vi "T1T2占空比副本.vi"() -> ()   [LabVIEW 2020]
uses:
  <vilib>/DAQmx/read.llb/DAQmx Read (Counter 1D DBL 1Chan NSamp).vi
  Global_Variable/Global.vi
  <vilib>/DAQmx/create/channels.llb/DAQmx Create Channel (CI-Period).vi
  <vilib>/DAQmx/configure/timing.llb/DAQmx Timing (Implicit).vi
  <vilib>/DAQmx/miscellaneous.llb/DAQmx Fill In Error Info.vi
  <userlib>/_MGI/1D Array/MGI Average/MGI Average (DBL[]).vi
  <vilib>/DAQmx/create/channels.llb/DAQmx Create Channel (CI-Pulse Width).vi
  <resource>/objmgr/daqmx.rc
panel:
  out "T2":dbl
  out "T2周期":dbl
  out "T1周期":dbl
  out "T1":dbl
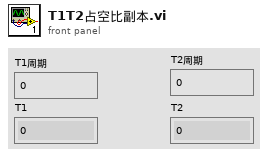
[diagram p1: front panel]
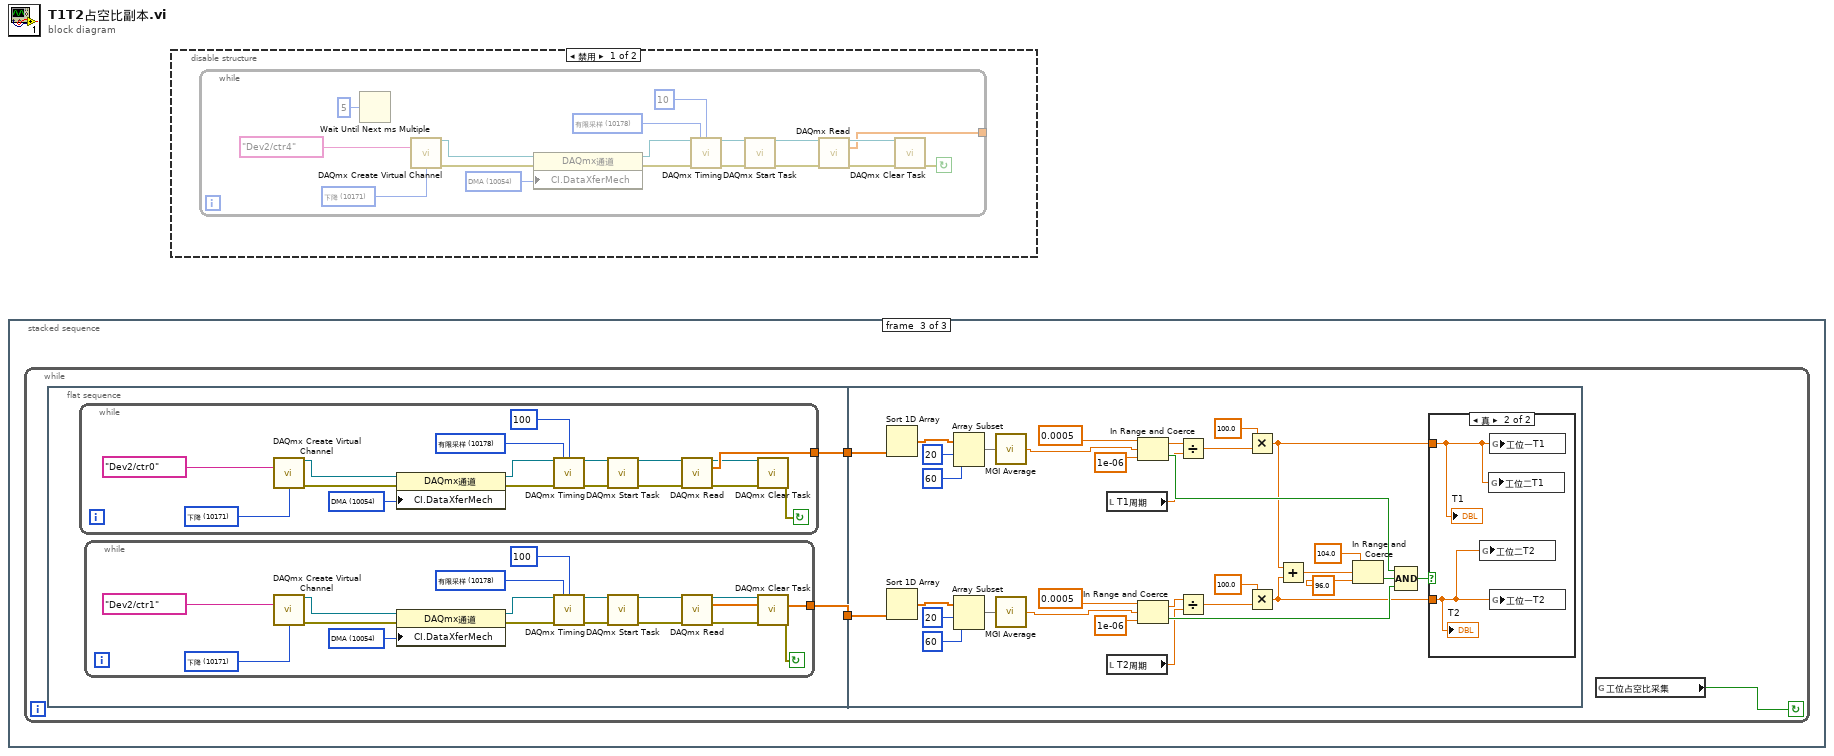
[diagram p0: block diagram]
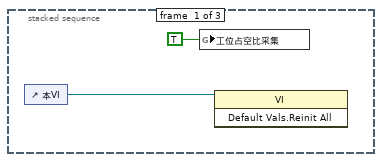
[diagram p3: hidden frame]
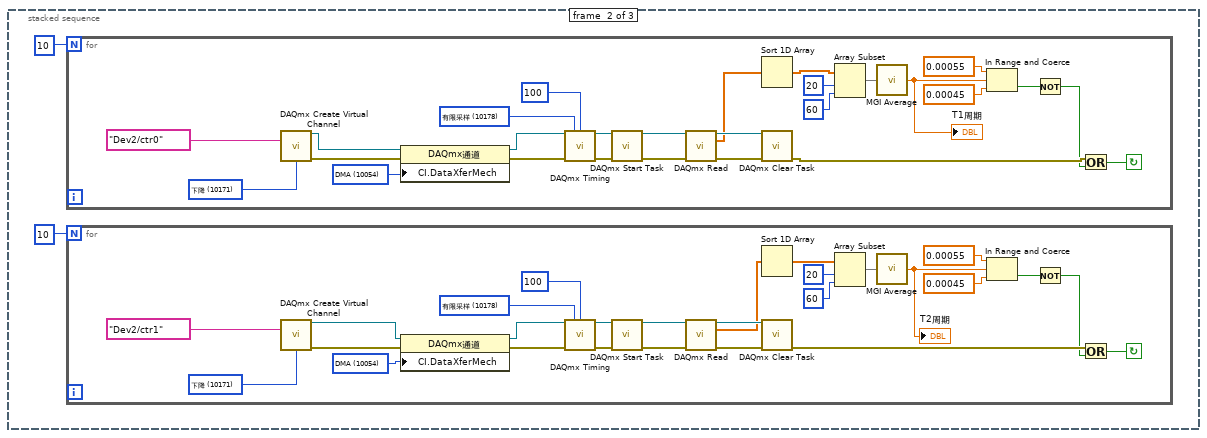
[diagram p4: hidden frame]
diagram:
  n1 = stacked-sequence {
    frame #0 {
      n2 = control-ref of="本VI"() -> (w2:refnum<vi>)
      n3 = global write "Global.vi" "工位占空比采集"(TRUE ("工位一占空比采集")) -> ()
      n4 = invoke class="VI" method="Default Vals.Reinit All"(reference=w2) -> ()  [unwired: 2 in, 3 out]
    }
    frame #1 {
      n5 = for {
        N: 10 -> [_]
        stop <- w32 continue-if-true
        w45 = 10054 items=["DMA"=10054, "中断"=10204, "程序控制I/O"=10264, "USB Bulk"=12590] ("CI.DataXferMech")
        w49 = 10178 items=["有限采样"=10178, "连续采样"=10123, "硬件定时单点"=12522] ("sample mode")
        w58 = 10171 items=["上升"=10280, "下降"=10171] ("starting edge")
        n6 = call-poly <vilib>:"DAQmx Create Virtual Channel.vi"("counter"=tag "Dev2/ctr0", "starting edge"=w58) -> ("task out"=w57:refnum<k21>, "error out"=w47:errorcluster)  [unwired: 12 in]
        n7 = property class="DAQmx通道"(reference=w57, error in=w47, "CI.DataXferMech"=w45) -> (reference out=w48:refnum<k21>, error out=w46:errorcluster)
        n8 = call-poly <vilib>:"DAQmx Timing.vi"("task/channels in"=w48, "sample mode"=w49, "samples per channel"=100, "error in"=w46) -> ("task out"=w56:refnum<k21>, "error out"=w55:errorcluster)  [unwired: 10 in]
        n9 = call <vilib>:"DAQmx Start Task.vi"("task/channels in"=w56, "error in"=w55) -> ("task out"=w54:refnum<k21>, "error out"=w53:errorcluster)  [unwired: 12 in]
        n10 = call-poly <vilib>:"DAQmx Read.vi"("task/channels in"=w54, "error in"=w53) -> ("task out"=w51:refnum<k21>, "data"=w39:dbl[], "error out"=w52:errorcluster)  [unwired: 11 in]
        n11 = Sort 1D Array(array=w39) -> (sorted array=w42:dbl[])
        n12 = call <vilib>:"DAQmx Clear Task.vi"("task in"=w51, "error in"=w52) -> ("error out"=w34:errorcluster)  [unwired: 13 in]
        n13 = Array Subset(array=w42, index=20 ("索引"), length=60 ("长度")) -> (w43:dbl[])
        n14 = call-poly <userlib>:"MGI Average.vi"("Double[]"=w43) -> ("Average"=w38:dbl)  [unwired: 1 in]
        "T1周期" <- w38
        n15 = In Range and Coerce(upper limit=0.00055 ("上限"), x=w38, lower limit=0.00045 ("上限")) -> (In Range?=w35:bool)  [unwired: 1 out]
        n16 = Not(x=w35) -> (.not. x?=w33:bool)
        n17 = Or(x=w34, y=w33) -> (x .or. y?=w32:bool)
      }
      n18 = for {
        N: 10 -> [_]
        stop <- w5 continue-if-true
        w18 = 10054 items=["DMA"=10054, "中断"=10204, "程序控制I/O"=10264, "USB Bulk"=12590] ("CI.DataXferMech")
        w22 = 10178 items=["有限采样"=10178, "连续采样"=10123, "硬件定时单点"=12522] ("sample mode")
        w31 = 10171 items=["上升"=10280, "下降"=10171] ("starting edge")
        n19 = call-poly <vilib>:"DAQmx Create Virtual Channel.vi"("counter"=tag "Dev2/ctr1", "starting edge"=w31) -> ("task out"=w30:refnum<k21>, "error out"=w20:errorcluster)  [unwired: 12 in]
        n20 = property class="DAQmx通道"(reference=w30, error in=w20, "CI.DataXferMech"=w18) -> (reference out=w21:refnum<k21>, error out=w19:errorcluster)
        n21 = call-poly <vilib>:"DAQmx Timing.vi"("task/channels in"=w21, "sample mode"=w22, "samples per channel"=100, "error in"=w19) -> ("task out"=w29:refnum<k21>, "error out"=w28:errorcluster)  [unwired: 10 in]
        n22 = call <vilib>:"DAQmx Start Task.vi"("task/channels in"=w29, "error in"=w28) -> ("task out"=w27:refnum<k21>, "error out"=w26:errorcluster)  [unwired: 12 in]
        n23 = call-poly <vilib>:"DAQmx Read.vi"("task/channels in"=w27, "error in"=w26) -> ("task out"=w24:refnum<k21>, "data"=w12:dbl[], "error out"=w25:errorcluster)  [unwired: 11 in]
        n24 = Sort 1D Array(array=w12) -> (sorted array=w16:dbl[])
        n25 = call <vilib>:"DAQmx Clear Task.vi"("task in"=w24, "error in"=w25) -> ("error out"=w8:errorcluster)  [unwired: 13 in]
        n26 = Array Subset(array=w16, index=20 ("索引"), length=60 ("长度")) -> (w15:dbl[])
        n27 = call-poly <userlib>:"MGI Average.vi"("Double[]"=w15) -> ("Average"=w9:dbl)  [unwired: 1 in]
        "T2周期" <- w9
        n28 = In Range and Coerce(upper limit=0.00055 ("上限"), x=w9, lower limit=0.00045 ("上限")) -> (In Range?=w7:bool)  [unwired: 1 out]
        n29 = Not(x=w7) -> (.not. x?=w6:bool)
        n30 = Or(x=w8, y=w6) -> (x .or. y?=w5:bool)
      }
    }
    frame #2 {
      n31 = while {
        stop <- w61 continue-if-true
        n32 = flat-sequence {
          tunnel: [w63] -> w60
          tunnel: [w62] -> w59
          tunnel: w60 -> [w98]
          tunnel: w59 -> [w101]
          frame #0 {
            n33 = while {
              tunnel: [w97] -> w63
              stop <- w81 continue-if-true
              w83 = 10054 items=["DMA"=10054, "中断"=10204, "程序控制I/O"=10264, "USB Bulk"=12590] ("CI.DataXferMech")
              w87 = 10178 items=["有限采样"=10178, "连续采样"=10123, "硬件定时单点"=12522] ("sample mode")
              w96 = 10171 items=["上升"=10280, "下降"=10171] ("starting edge")
              n34 = call-poly <vilib>:"DAQmx Create Virtual Channel.vi"("counter"=tag "Dev2/ctr0", "starting edge"=w96) -> ("task out"=w95:refnum<k21>, "error out"=w85:errorcluster)  [unwired: 12 in]
              n35 = property class="DAQmx通道"(reference=w95, error in=w85, "CI.DataXferMech"=w83) -> (reference out=w86:refnum<k21>, error out=w84:errorcluster)
              n36 = call-poly <vilib>:"DAQmx Timing.vi"("task/channels in"=w86, "sample mode"=w87, "samples per channel"=100, "error in"=w84) -> ("task out"=w94:refnum<k21>, "error out"=w93:errorcluster)  [unwired: 10 in]
              n37 = call <vilib>:"DAQmx Start Task.vi"("task/channels in"=w94, "error in"=w93) -> ("task out"=w92:refnum<k21>, "error out"=w91:errorcluster)  [unwired: 12 in]
              n38 = call-poly <vilib>:"DAQmx Read.vi"("task/channels in"=w92, "error in"=w91) -> ("task out"=w89:refnum<k21>, "data"=w97:dbl[], "error out"=w90:errorcluster)  [unwired: 11 in]
              n39 = call <vilib>:"DAQmx Clear Task.vi"("task in"=w89, "error in"=w90) -> ("error out"=w81:errorcluster)  [unwired: 13 in]
            }
            n40 = while {
              tunnel: [w80] -> w62
              stop <- w64 continue-if-true
              w66 = 10054 items=["DMA"=10054, "中断"=10204, "程序控制I/O"=10264, "USB Bulk"=12590] ("CI.DataXferMech")
              w70 = 10178 items=["有限采样"=10178, "连续采样"=10123, "硬件定时单点"=12522] ("sample mode")
              w79 = 10171 items=["上升"=10280, "下降"=10171] ("starting edge")
              n41 = call-poly <vilib>:"DAQmx Create Virtual Channel.vi"("counter"=tag "Dev2/ctr1", "starting edge"=w79) -> ("task out"=w78:refnum<k21>, "error out"=w68:errorcluster)  [unwired: 12 in]
              n42 = property class="DAQmx通道"(reference=w78, error in=w68, "CI.DataXferMech"=w66) -> (reference out=w69:refnum<k21>, error out=w67:errorcluster)
              n43 = call-poly <vilib>:"DAQmx Timing.vi"("task/channels in"=w69, "sample mode"=w70, "samples per channel"=100, "error in"=w67) -> ("task out"=w77:refnum<k21>, "error out"=w76:errorcluster)  [unwired: 10 in]
              n44 = call <vilib>:"DAQmx Start Task.vi"("task/channels in"=w77, "error in"=w76) -> ("task out"=w75:refnum<k21>, "error out"=w74:errorcluster)  [unwired: 12 in]
              n45 = call-poly <vilib>:"DAQmx Read.vi"("task/channels in"=w75, "error in"=w74) -> ("task out"=w72:refnum<k21>, "data"=w80:dbl[], "error out"=w73:errorcluster)  [unwired: 11 in]
              n46 = call <vilib>:"DAQmx Clear Task.vi"("task in"=w72, "error in"=w73) -> ("error out"=w64:errorcluster)  [unwired: 13 in]
            }
          }
          frame #1 {
            n47 = Sort 1D Array(array=w98) -> (sorted array=w112:dbl[])
            n48 = Sort 1D Array(array=w101) -> (sorted array=w115:dbl[])
            n49 = Array Subset(array=w112, index=20 ("索引"), length=60 ("长度")) -> (w113:dbl[])
            n50 = Array Subset(array=w115, index=20 ("索引"), length=60 ("长度")) -> (w114:dbl[])
            n51 = call-poly <userlib>:"MGI Average.vi"("Double[]"=w113) -> ("Average"=w116:dbl)  [unwired: 1 in]
            n52 = call-poly <userlib>:"MGI Average.vi"("Double[]"=w114) -> ("Average"=w118:dbl)  [unwired: 1 in]
            n53 = local read "T1周期"() -> (w121:dbl)
            n54 = local read "T2周期"() -> (w122:dbl)
            n55 = In Range and Coerce(upper limit=0.0005 ("上限"), x=w116, lower limit=1e-06 ("上限")) -> (coerced(x)=w117:dbl, In Range?=w127:bool)
            n56 = In Range and Coerce(upper limit=0.0005 ("上限"), x=w118, lower limit=1e-06 ("上限")) -> (coerced(x)=w119:dbl, In Range?=w128:bool)
            n57 = Divide(x=w117, y=w121) -> (x/y=w120:dbl)
            n58 = Divide(x=w119, y=w122) -> (x/y=w123:dbl)
            n59 = Multiply(x=100.0, y=w120) -> (x*y=w124:dbl)
            n60 = Multiply(x=100.0, y=w123) -> (x*y=w125:dbl)
            n61 = Add(x=w124, y=w125) -> (x+y=w126:dbl)
            n62 = In Range and Coerce(upper limit=104.0 ("上限"), x=w126, lower limit=96.0 ("下限")) -> (In Range?=w129:bool)  [unwired: 1 out]
            n63 = Compound Arithmetic op=AND ("复合运算")(w127, w129, w128) -> (w130:bool)
            n64 = case shown="真" w130 {
              tunnel: w124 -> [_ w132]
              tunnel: w125 -> [_ w131]
              frame False {
              }
              frame True {
                n65 = global write "Global.vi" "工位二T2"(w131) -> ()
                n66 = global write "Global.vi" "工位二T1"(w132) -> ()
                n67 = global write "Global.vi" "工位一T1"(w132) -> ()
                n68 = global write "Global.vi" "工位一T2"(w131) -> ()
                "T1" <- w132
                "T2" <- w131
              }
            }
          }
        }
        n69 = global read "Global.vi" "工位占空比采集"() -> (w61:bool)
      }
    }
  }
  n70 = disable-structure shown="禁用" {
    frame Disabled {
      n71 = while {
        tunnel: [w140] -> _
        stop <- w134 continue-if-true
        w136 = 10054 items=["DMA"=10054, "中断"=10204, "程序控制I/O"=10264, "USB Bulk"=12590] ("CI.DataXferMech")
        w141 = 10178 items=["有限采样"=10178, "连续采样"=10123, "硬件定时单点"=12522] ("sample mode")
        w150 = 10171 items=["上升"=10280, "下降"=10171] ("starting edge")
        n72 = Wait Until Next ms Multiple(millisecond multiple=u32 5 ("毫秒倍数")) -> ()  [unwired: 1 out]
        n73 = call-poly <vilib>:"DAQmx Create Virtual Channel.vi"("counter"=tag "Dev2/ctr4", "starting edge"=w150) -> ("task out"=w149:refnum<k21>, "error out"=w138:errorcluster)  [unwired: 12 in]
        n74 = property class="DAQmx通道"(reference=w149, error in=w138, "CI.DataXferMech"=w136) -> (reference out=w139:refnum<k21>, error out=w137:errorcluster)
        n75 = call-poly <vilib>:"DAQmx Timing.vi"("task/channels in"=w139, "sample mode"=w141, "samples per channel"=10, "error in"=w137) -> ("task out"=w148:refnum<k21>, "error out"=w147:errorcluster)  [unwired: 10 in]
        n76 = call <vilib>:"DAQmx Start Task.vi"("task/channels in"=w148, "error in"=w147) -> ("task out"=w146:refnum<k21>, "error out"=w145:errorcluster)  [unwired: 12 in]
        n77 = call-poly <vilib>:"DAQmx Read.vi"("task/channels in"=w146, "error in"=w145) -> ("task out"=w143:refnum<k21>, "data"=w140:dbl[], "error out"=w144:errorcluster)  [unwired: 11 in]
        n78 = call <vilib>:"DAQmx Clear Task.vi"("task in"=w143, "error in"=w144) -> ("error out"=w134:errorcluster)  [unwired: 13 in]
      }
    }
    frame Enabled {
    }
  }
